vi "indicadores.vi"() -> ()   [LabVIEW 2016]
panel:
  out "Thermometer":cluster{dbl, dbl}(slide)={0.0, -0.5510204081632654} scale=-3.0..3.0
  out "Gauge":cluster{dbl, dbl}(knob)={0.0, 3.0} scale=-3.0..3.0
  in  "Stop Button":bool
  out "Waveform Chart":cluster{dbl, dbl, dbl, dbl}(graph)
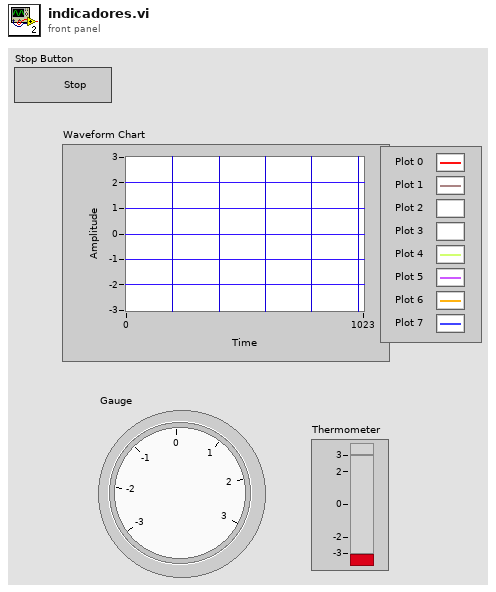
[diagram p1: front panel]
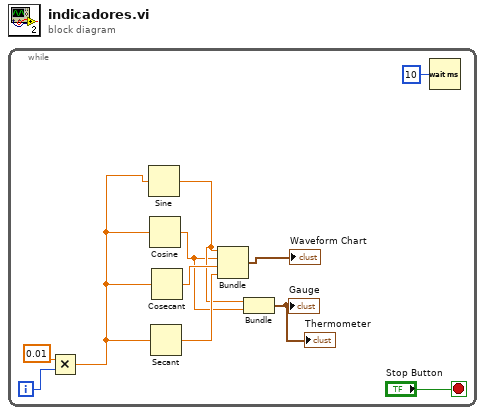
[diagram p0: block diagram]
diagram:
  n1 = while {
    i -> [w10]
    stop <- "Stop Button" stop-if-true
    n2 = Multiply(x=0.01, y=w10) -> (x*y=w8:dbl)
    n3 = Sine(x=w8) -> (sin(x)=w3:dbl)
    n4 = Cosine(x=w8) -> (cos(x)=w2:dbl)
    n5 = Secant(1:w8) -> (0:w5:dbl)
    n6 = Cosecant(1:w8) -> (0:w6:dbl)
    n7 = Bundle(w3, w2, w6, w5) -> (→"Waveform Chart":cluster{dbl, dbl, dbl, dbl})  [unwired: 1 in]
    n8 = Bundle(w3, w2) -> (→"Gauge" →"Thermometer":cluster{dbl, dbl})  [unwired: 1 in]
    n9 = Wait (ms)(milliseconds to wait=u32 10) -> ()  [unwired: 1 out]
  }
